vi "Batch Axis Shift.vi"(8 "Offsets In":dbl[][](array[numeric]), 9 "Coordinate Switch":bool, 10 "Data In":dbl[][](array[numeric]), 11 "Direction":enum16{" +", " - "}(ring)) -> (2 "Data Out":dbl[][](array[numeric]) caption="LBCB 1 Data")   [LabVIEW 2013]
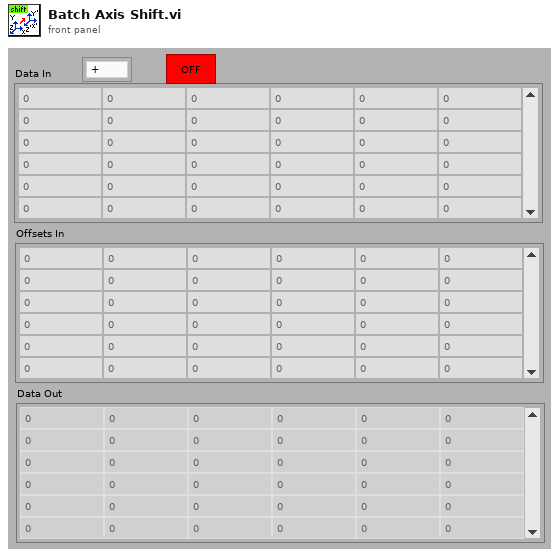
[diagram p1: front panel]
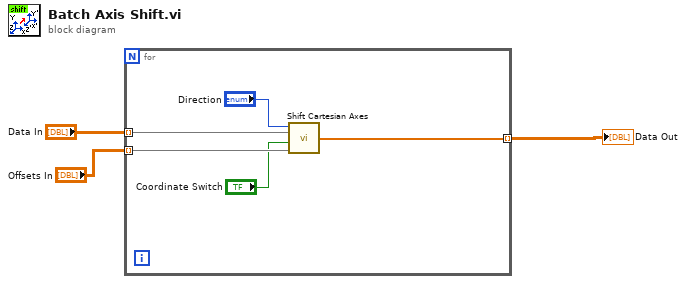
[diagram p0: block diagram]
diagram:
  n1 = for {
    tunnel: "Data In" -> [w8] mode=indexing
    tunnel: "Offsets In" -> [w7] mode=indexing
    tunnel: [w6] -> w1 mode=indexing
    n2 = call "Shift Cartesian Axes.vi"("Coordinate Offset"=w7, "Coordinate Switch"="Coordinate Switch", "Coordinate Input"=w8, "Direction"="Direction") -> ("Coordinate Output"=w6:dbl[])
  }
  "Data Out" <- w1
